vi "Find Cameras.vi"(4 "error in (no error)":errorcluster, 7 "cameraCount":i32) -> (0 "error out":errorcluster, 2 "function return":i32, 3 "cameraCount out":i32)   [LabVIEW 2020, in "ThorConfocal.lvlib"]
doc: "long FindCameras(long &cameraCount);"
uses:
  ThorConfocal.lvlib
  C:/Program Files/Thorlabs/ThorImageLS 4.1/Modules_Native/ThorConfocal.dll
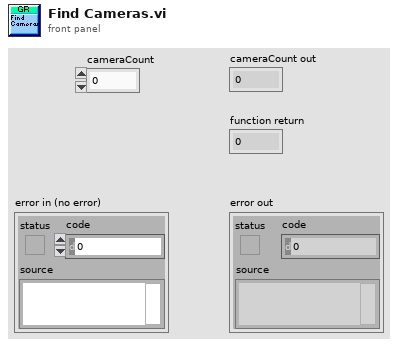
[diagram p1: front panel]
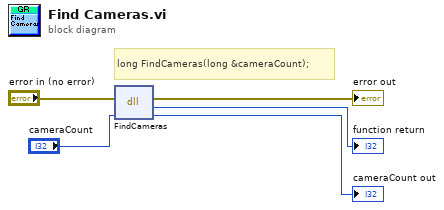
[diagram p0: block diagram]
diagram:
  # "long FindCameras(long &cameraCount);"
  n1 = dll-call lib="C:/Program Files/Thorlabs/ThorImageLS 4.1/Modules_Native/ThorConfocal.dll" fn="FindCameras"(error in="error in (no error)", "cameraCount"="cameraCount") -> (error out=→"error out":errorcluster, "return type"=→"function return":i32, "cameraCount"=→"cameraCount out":i32)  [unwired: 2 in, 1 out]
